vi "Hide Animated Busy Icon.vi"(2 "Error In":errorcluster) -> (7 "Error Out":errorcluster)   [LabVIEW 2019]
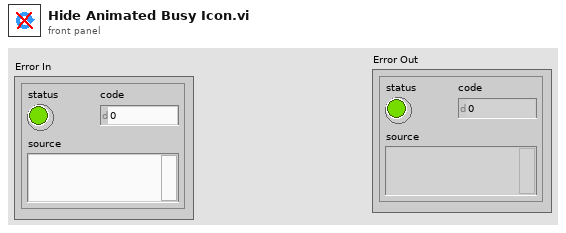
[diagram p1: front panel]
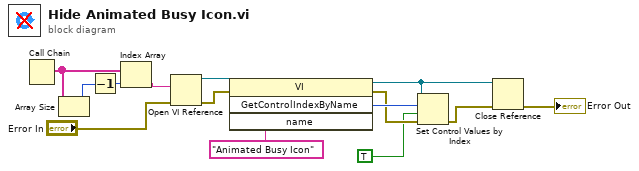
[diagram p0: block diagram]
diagram:
  n1 = Call Chain() -> (call chain=w14:string[])
  n2 = Array Size(array=w14) -> (size(s)=w13:i32)
  n3 = Decrement(x=w13) -> (x-1=w12:i32)
  n4 = Index Array(array=w14, index=w12) -> (element=w11:string)
  n5 = Open VI Reference(vi path=w11, error in (no error)="Error In") -> (vi reference=w6:refnum<vi>, error out=w5:errorcluster)  [unwired: 4 in]
  n6 = invoke class="VI" method="GetControlIndexByName"(reference=w6, error in=w5, "name"="Animated Busy Icon" ("element")) -> (reference out=w3:refnum<vi>, error out=w8:errorcluster, "GetControlIndexByName"=w9:i32)  [unwired: 1 in, 1 out]
  n7 = Set Control Values by Index(0:w3, 1:w9, 2:TRUE, 3:w8) -> (11:w7:errorcluster)
  n8 = Close Reference(reference=w3, error in (no error)=w7) -> (error out=→"Error Out":errorcluster)
